vi "Write Time Scale.vi"(8 "error in (no error)":errorcluster, 10 "Time Scale [ms]":u32, 11 "Cashier In":refnum<class "Cashier.lvclass">) -> (0 "error out":errorcluster, 3 "Cashier Out":refnum<class "Cashier.lvclass">)   [LabVIEW 2020, in "Cashier.lvclass"]
uses:
  Cashier.lvclass
  Cashier.lvclass/Cashier.ctl
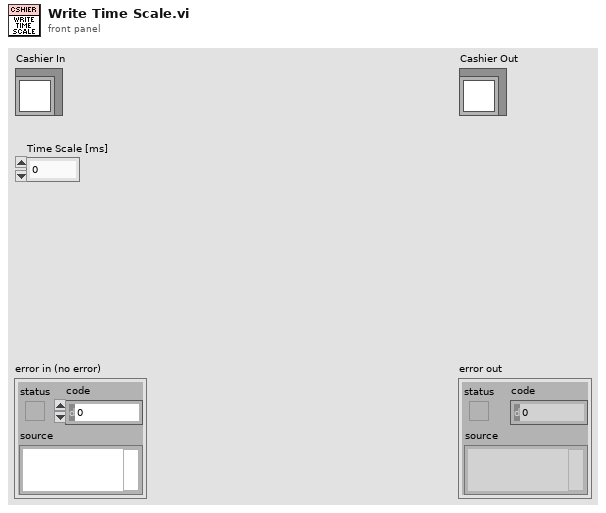
[diagram p1: front panel]
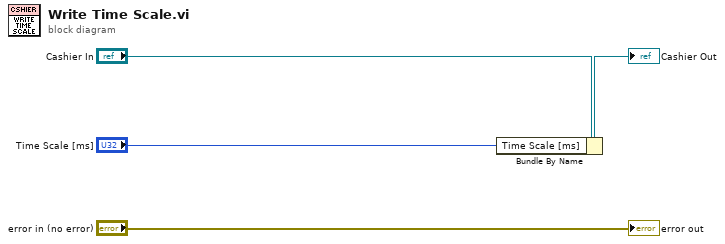
[diagram p0: block diagram]
diagram:
  n1 = Bundle By Name(cluster="Cashier In", "Time Scale [ms]"="Time Scale [ms]") -> (→"Cashier Out":refnum<class "Cashier.lvclass">)
  "error out" <- "error in (no error)"
